vi "FlexDDS-NG_DCP_WriteRegAD9910.vi"(8 "register content":u64 format="%x", 9 "AD9910 register name":string="STP0", 10 "Channels":T1(ring)=enum."Both channels", 11 "initial instruction string":string) -> (3 "appended instruction string":string)   [LabVIEW 2016]
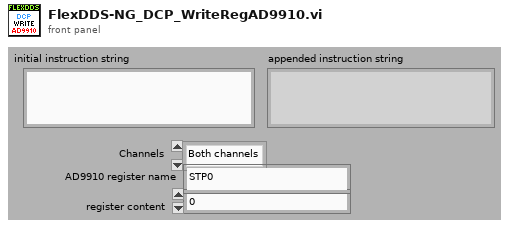
[diagram p1: front panel]
types:
  T1 = enum32{"Channel 0", "Channel 1", "Both channels"}
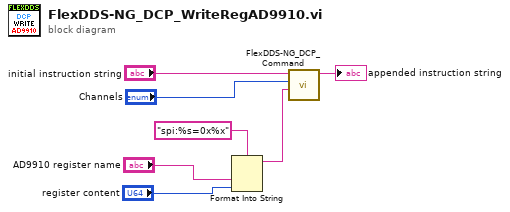
[diagram p0: block diagram]
diagram:
  n1 = Format Into String(format string="spi:%s=0x%x", "AD9910 register name", "register content") -> (resulting string=w1:string)  [unwired: 2 in, 1 out]
  n2 = call "FlexDDS-NG_DCP_Command.vi"("command string"=w1, "Channels"="Channels", "initial instruction string"="initial instruction string") -> ("appended instruction string"=→"appended instruction string":string)  [unwired: 8 in]
